vi "Generate logfile.vi"(6 "Normál mérés?":bool, 8 "error in":errorcluster, 9 "Tem Log file path":path, 10 "Log file path":path, 11 "MulticolumnListbox in":refnum<vi>) -> (0 "error out":errorcluster)   [LabVIEW 2014]
uses:
  <vilib>/Utility/file.llb/Write To Spreadsheet File (string).vi
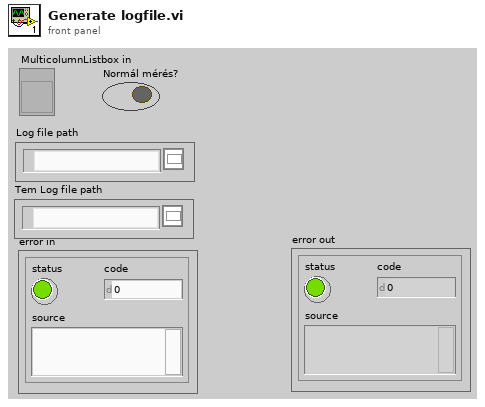
[diagram p1: front panel]
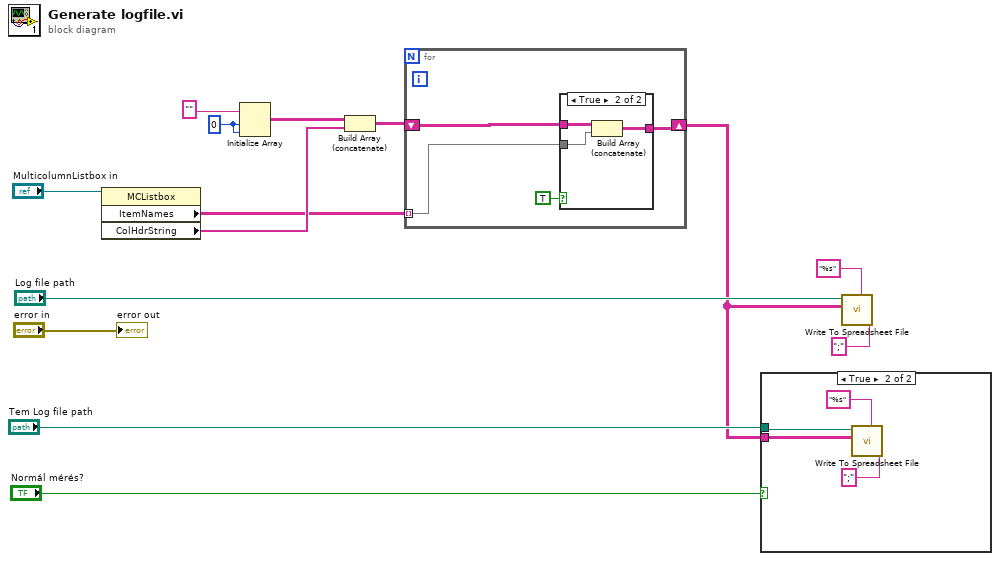
[diagram p0: block diagram]
diagram:
  w12 = 0 ("dimension size")
  n1 = property class="MCListbox"(reference="MulticolumnListbox in") -> ("ItemNames"=w8:string[][], "ColHdrString"=w9:string[])  [unwired: 1 in, 2 out]
  n2 = Initialize Array("" ("delimiter (Tab)"), w12, w12) -> (w11:string[][])
  n3 = Build Array (concatenate)(w11, w9) -> (w10:string[][])
  n4 = for {
    tunnel: w8 -> [w18] mode=indexing
    shift-right: [w16] -> w1
    shift-left: w10 -> [w17]
    n5 = case shown="True" TRUE {
      tunnel: w18 -> [_ w21]
      tunnel: w17 -> [w19 w22]
      tunnel: [w19 w20] -> w16
      frame False {
      }
      frame True {
        n6 = Build Array (concatenate)(w22, w21) -> (w20:string[][])
      }
    }
  }
  n7 = case shown="True" "Normál mérés?" {
    tunnel: "Tem Log file path" -> [_ w24]
    tunnel: w1 -> [_ w23]
    frame False {
    }
    frame True {
      n8 = call-poly <vilib>:"Write To Spreadsheet File.vi"("delimiter (\\t)"=";" ("delimiter (\\t)"), "format (%s)"="%s" ("format (%.3f)"), "2D data"=w23, "file path (dialog if empty)"=w24) -> ()  [unwired: 4 in, 1 out]
    }
  }
  n9 = call-poly <vilib>:"Write To Spreadsheet File.vi"("delimiter (\\t)"=";" ("delimiter (\\t)"), "format (%s)"="%s" ("format (%.3f)"), "2D data"=w1, "file path (dialog if empty)"="Log file path") -> ()  [unwired: 4 in, 1 out]
  "error out" <- "error in"
